vi "configuration UI.vi"() -> ()   [LabVIEW 2018, in "TDMS datalogger editor node.lvclass"]
uses:
  TDMS datalogger editor node.lvclass
  <vilib>/NI/Configuration Framework/Node/NodeRef.ctl
  <vilib>/NI/Configuration Framework/Node/NISE_CEF_Node.lvclass
  <vilib>/NI/AMC/Message Queue.ctl
  <vilib>/NI/AMC/Message.ctl
  <vilib>/NI/Tools/Keyed Array/KeyedArray.ctl
  <vilib>/NI/Configuration Framework/Node/UserEventRef.ctl
  <vilib>/NI/Configuration Framework/Controls/EventCluster.ctl
  <vilib>/NI/DCAF UI Toolkit/Controls/Move One Right.ctl
  <vilib>/NI/DCAF UI Toolkit/Controls/Move All Right.ctl
  <vilib>/NI/DCAF UI Toolkit/Controls/Move One Left.ctl
  <vilib>/NI/Configuration Framework/Node/NodeChangeEvent.ctl
  <vilib>/NI/DCAF UI Toolkit/Controls/Add.ctl
  <vilib>/NI/DCAF UI Toolkit/Controls/Remove.ctl
  <vilib>/NI/Configuration Framework/Node/RefreshUIEvent.ctl
  <vilib>/NI/Configuration Framework/Node/StopEvent.ctl
  <vilib>/NI/Configuration Framework/Node/CacheState.ctl
  <vilib>/NI/DCAF/Tag Editor Core/Table API/Available Tag Menu/channel action event.ctl
  <vilib>/NI/DCAF/Tag Editor Core/Table API/Available Tag Menu/dialog output action.ctl
  <vilib>/NI/Tag Bus Module Framework/channel/TBM channel.lvclass
  <vilib>/NI/Tag Bus/tag/tag descriptor.lvclass
  <vilib>/NI/DCAF/Tag Editor Core/Table API/Table Manager/Call Back Ref Type Def.ctl
  <vilib>/NI/DCAF/Tag Editor Core/Configuration Editor/Classes/Engine Parent/Engine Parent Editor Node.lvclass
  <vilib>/NI/DCAF/Tag Editor Core/Configuration Editor/Classes/Module editor node/module editor node.lvclass
  <vilib>/NI/DCAF UI Toolkit/Controls/Configure.ctl
  <vilib>/NI/DCAF/Tag Editor Core/Table API/Table Manager/object ref.ctl
  <vilib>/NI/DCAF/Tag Editor Core/Table API/Table Manager/references.ctl
  Control Refs.ctl
  <vilib>/Utility/miscctls.llb/LVPositionTypeDef.ctl
  <vilib>/NI/DCAF/Tag Editor Core/Table API/Listbox/Multi Column Listbox.lvclass
  <vilib>/NI/Configuration Framework/NISE_CEF_TreeControl.lvlib
  <vilib>/NI/DCAF UI Toolkit/Controls/DCAF UI Elements.lvlib
  <vilib>/NI/Tools/Keyed Array/Tools_KeyedArray.lvlib
  <vilib>/NI/AMC/AMC.lvlib
  <vilib>/NI/DCAF/Tag Editor Core/Table API/Table Manager/Table Manager.lvclass
  <vilib>/NI/DCAF/Tag Editor Core/Table API/Table Manager.lvlib
panel:
  in  "References":T1
  in  "user event out":refnum<user-event>
  in  "cache state":T2
  in  "stop event":T3
  in  "refresh UI":T4
  in  "node change":T5
  in  "Tab Control":T6(tab)
  in  "channels":i32(listbox)
  in  "remove":T7
  in  "avail tags":i32(listbox)=-1
  in  "add all":T8
  in  "add1":T9
  in  "Use Dynamic File Name":bool
  out "Logging File Path":string
  in  "file name error":bool
  in  "Log Directory":string
  in  "File Name":string
  out "Enable Tag":string
  in  "path error":bool
  in  "Use Enable Channel":bool
  in  "recalc":bool
  out "Approximate Memory Usage":dbl
  in  "Queue Size":u16=2
  in  "Scans Per Write":u16=20
  in  "Log Directory":path
  out "Dynamic File Name Tag":string
  in  "Maximum Age of Files (days)":dbl=365.0
  in  "Rotate count":u32 caption="Maximum Number of Archived Files To Keep"
  in  "archive in place":bool caption="Archive Old Logs in Original Directory"
  in  "Archive Directory":string
  in  "Archive Directory":path
  in  "archive error":bool
  in  "Maximum File Size (KB)":i64=10000
  in  "Channel Subscription Pattern Matches":string[](array[string])
  in  "Enable Dynamic Mapping":bool
  in  "Remove Group":T10
  in  "Add Group":T11
  in  "Remove from Group":T9
  in  "Add to Group":T7
  in  "avail logged tags":i32(listbox)=-1
  in  "Groups":string(tree)="Channel1"
  in  "Add Group Name":string caption="File Name"
  in  "File Property Settings":T12
  in  "File Properties":i32(listbox)=-1
  in  "Add File Property":T11
  in  "Remove File Property":T10
  in  "user event":T13
  in  "main queue":T14
  in  "node ref":T15
  # "kB"
  # "Note: This value ignores dynamic mapping"
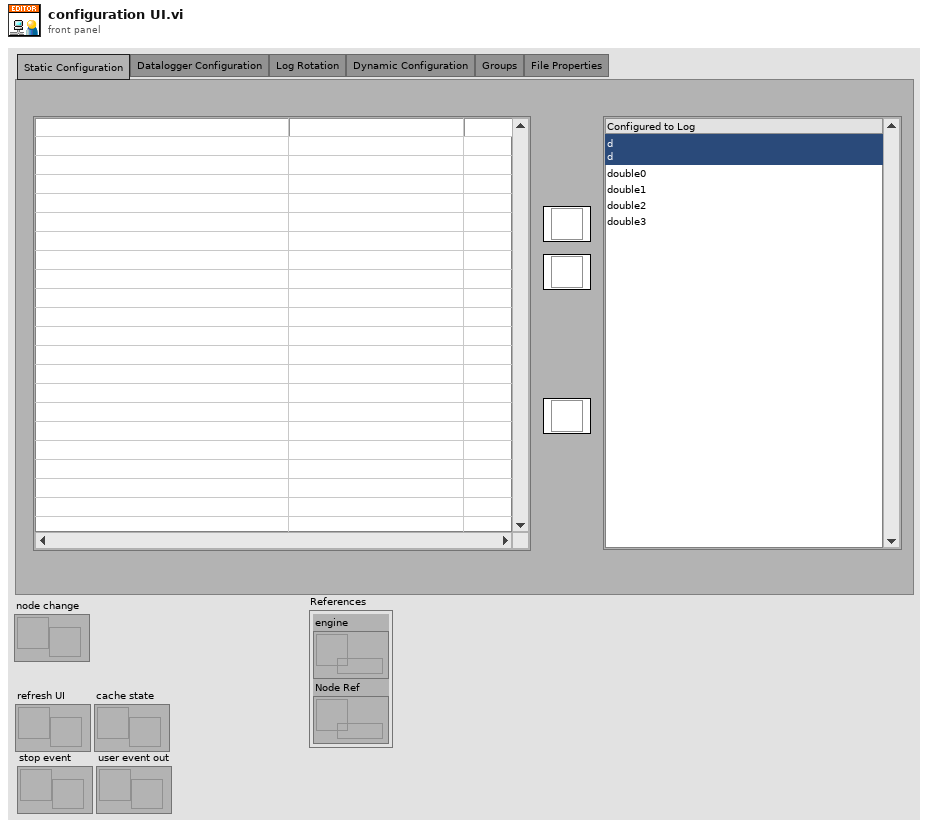
[diagram p1: front panel]
types:
  T1 = typedef "Table Manager.lvlib/Table Manager.lvclass/object ref.ctl" = cluster{"engine":refnum<data-value>, "Node Ref":refnum<data-value>}
  T2 = typedef "NISE_CEF_Node.lvclass/CacheState.ctl" = refnum<user-event>
  T3 = typedef "NISE_CEF_Node.lvclass/StopEvent.ctl" = refnum<user-event>
  T4 = typedef "NISE_CEF_Node.lvclass/RefreshUIEvent.ctl" = refnum<user-event>
  T5 = typedef "NISE_CEF_Node.lvclass/NodeChangeEvent.ctl" = refnum<user-event>
  T6 = enum32{"Static Configuration", "Datalogger Configuration", "Log Rotation", "Dynamic Configuration", "Groups", "File Properties"}
  T7 = typedef "DCAF UI Elements.lvlib/Move One Left.ctl" = bool
  T8 = typedef "DCAF UI Elements.lvlib/Move All Right.ctl" = bool
  T9 = typedef "DCAF UI Elements.lvlib/Move One Right.ctl" = bool
  T10 = typedef "DCAF UI Elements.lvlib/Remove.ctl" = bool
  T11 = typedef "DCAF UI Elements.lvlib/Add.ctl" = bool
  T12 = typedef "DCAF UI Elements.lvlib/Configure.ctl" = bool
  T13 = typedef "NISE_CEF_Node.lvclass/UserEventRef.ctl" = refnum<user-event>
  T14 = typedef "AMC.lvlib/Message Queue.ctl" = refnum<queue>
  T15 = typedef "NISE_CEF_Node.lvclass/NodeRef.ctl" = refnum<data-value>
  T16 = typedef "Control Refs.ctl" = cluster{"avail tags ref":refnum<vi>, "channels ref":refnum<vi>, "File Name ref":refnum<vi>, "Win Log Dir ref":refnum<vi>, "Linux Log Dir ref":refnum<vi>, "Scans Per Write ref":refnum<vi>, "Queue Size ref":refnum<vi>, "Use Enable Channel ref":refnum<vi>, "Maximum File Size ref":refnum<vi>, "Rotate Count ref":refnum<vi>, "Archive in Place ref":refnum<vi>, "Win Archive Dir ref":refnum<vi>, "Linux Archive Dir ref":refnum<vi>, "Max Age ref":refnum<vi>, "Enable Dynamic Mapping ref":refnum<vi>, "Channel Subscription Pattern Matches ref":refnum<vi>, "Add Group Name ref":refnum<vi>, "Groups ref":refnum<vi>, "avail logged tags ref":refnum<vi>, "Archive Error ref":refnum<vi>, "path error ref":refnum<vi>, "file name error ref":refnum<vi>, "Logging File Path":refnum<vi>}
  T17 = typedef "Table Manager.lvlib/Table Manager.lvclass/references.ctl" = cluster{"stop event":T3, "refresh UI":T4, "cache state":T2, "node change":T5, "user event out":refnum<user-event>, "main queue":T14, "user event":T13}
  T18 = typedef "LVPositionTypeDef.ctl" = cluster{"Left":i32, "Top":i32}
  T19 = typedef "Table Manager.lvlib/Column.lvclass/Column Descriptor.ctl" = cluster{"name":string, "caption":string, "Column Type":T20, "Params":string, "AutoSizeMode":i32, "FillWeight":sgl, "MinWidth":u32, "tooltip":string, "Enum Reference":refnum<vi>, "Channel suffix":string, "Read Only":bool, "Call Back VI":T21, "DT Dependency":i32, "name dependency":i32, "data type":T22, "Custom Column":refnum<class "Column.lvclass">}
  T20 = typedef "Table Manager.lvlib/Column.lvclass/Column Type.ctl" = enum16{"String", "Mapping", "Enum", "Custom"}
  T21 = typedef "Table Manager.lvlib/Table Manager.lvclass/Call Back Ref Type Def.ctl" = refnum<vi>
  T22 = typedef "tag bus.lvlib/tag descriptor.lvclass/Data Type.ctl" = enum16{"Double", "Single", "I64", "I32", "I16", "I8", "U64", "U32", "U16", "U8", "Boolean", "String", "Array of Double", "Array of Single", "Array of I64", "Array of I32", "Array of I16", "Array of I8", "Array of U64", "Array of U32", "Array of U16", "Array of U8", "Array of Boolean", "Array of String"}
  T23 = typedef "Table Manager.lvlib/Table Manager.lvclass/Table Events.ctl" = cluster{"Menu Selection":refnum<user-event>}
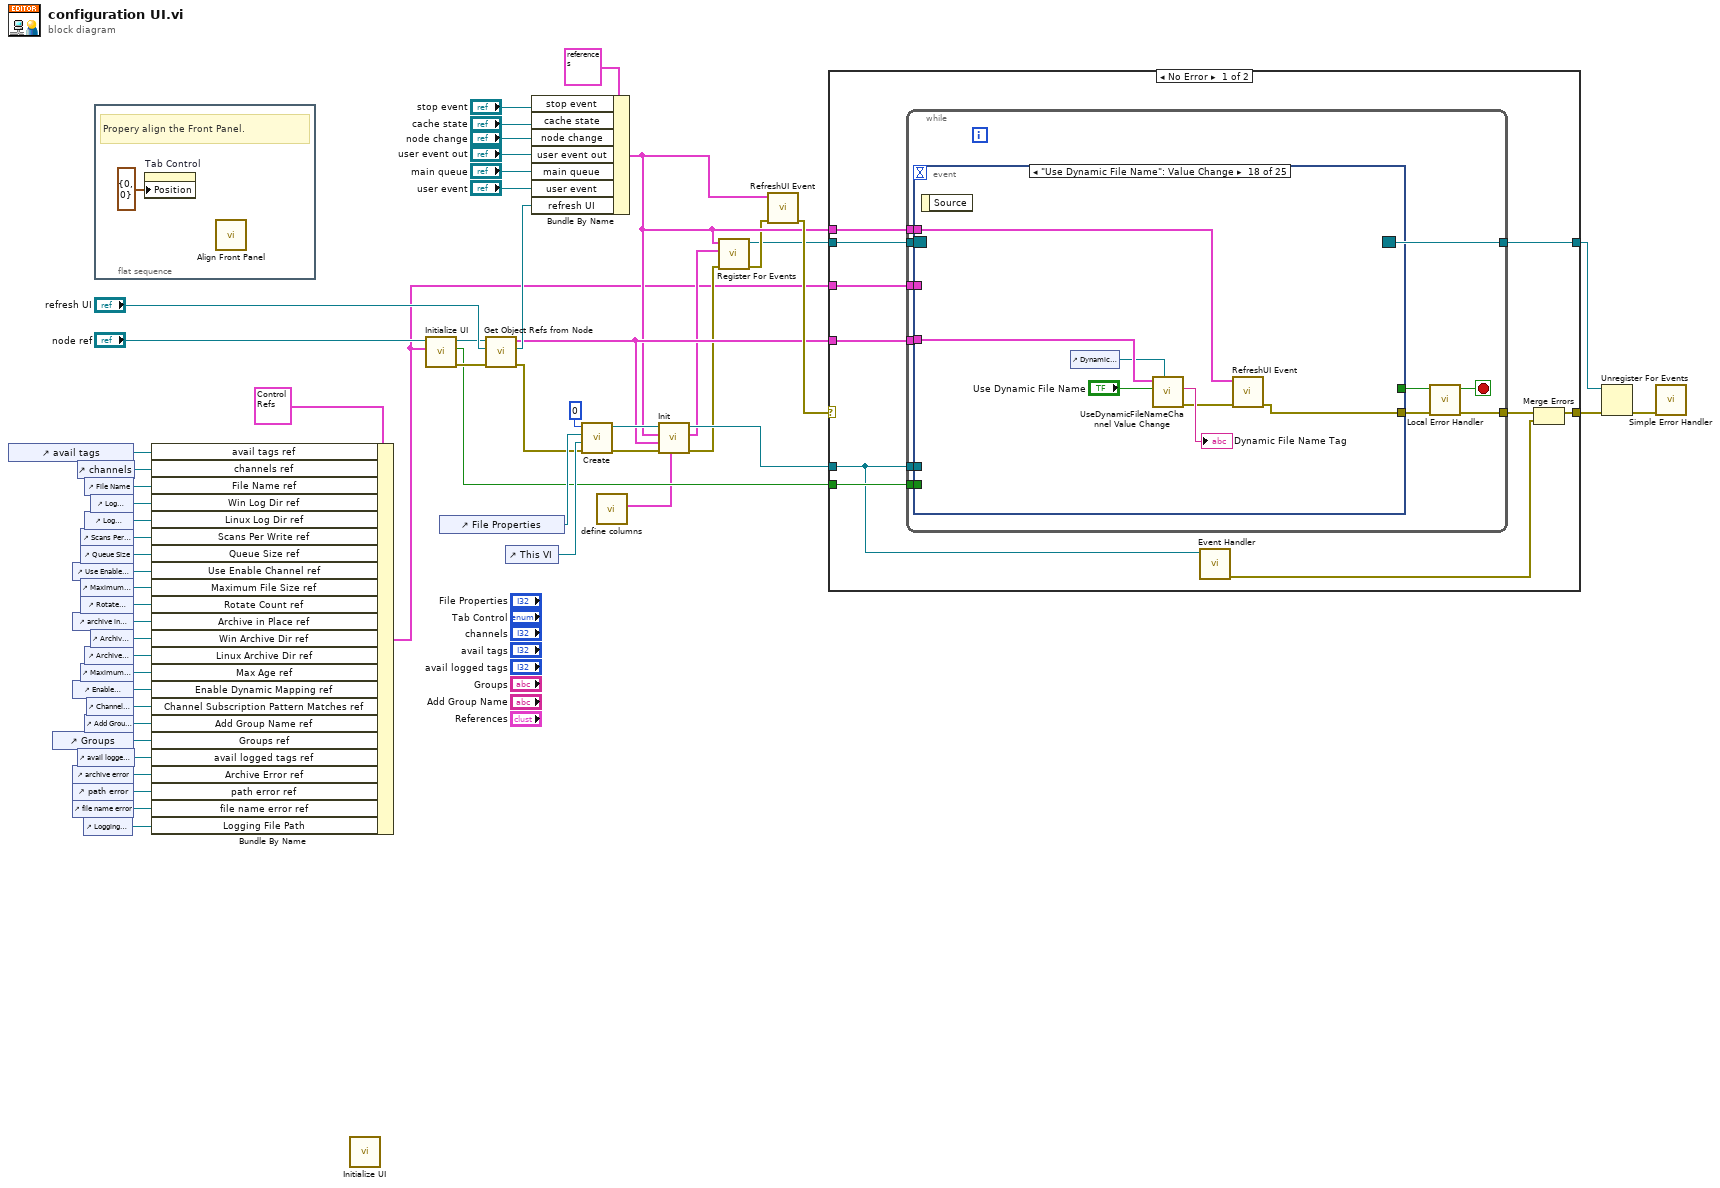
[diagram p0: block diagram]
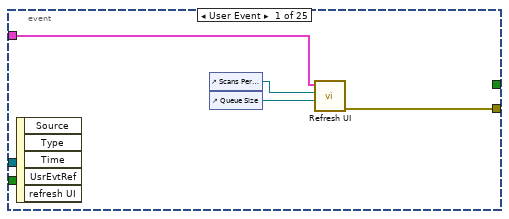
[diagram p2: hidden frame]
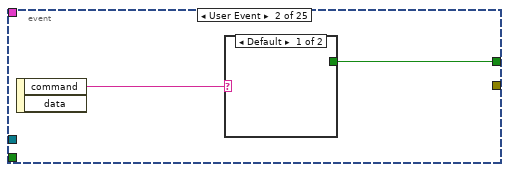
[diagram p3: hidden frame]
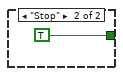
[diagram p4: hidden frame]
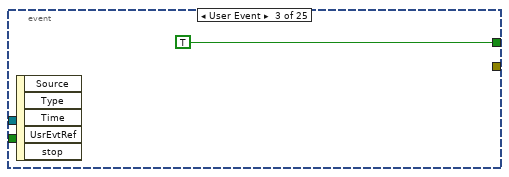
[diagram p5: hidden frame]
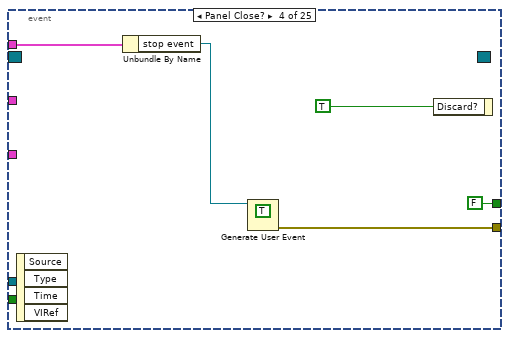
[diagram p6: hidden frame]
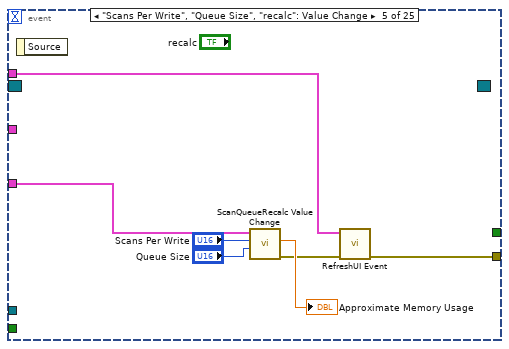
[diagram p7: hidden frame]
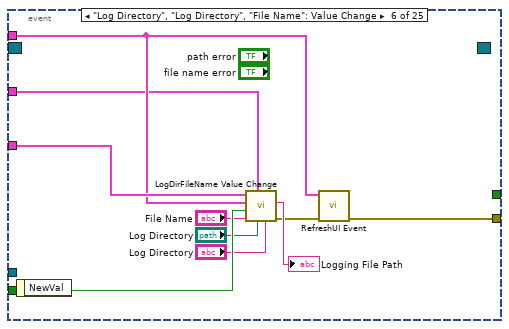
[diagram p8: hidden frame]
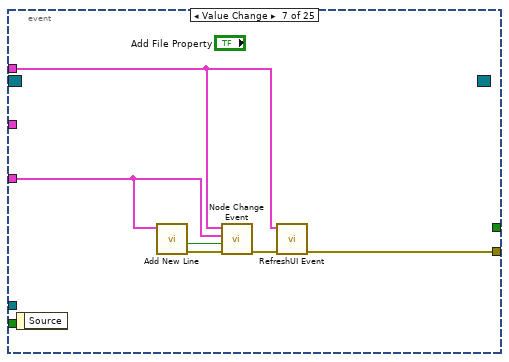
[diagram p9: hidden frame]
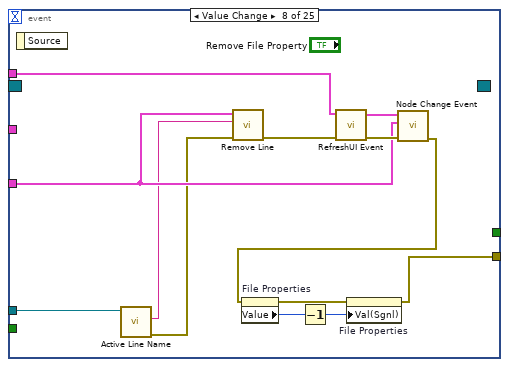
[diagram p10: hidden frame]
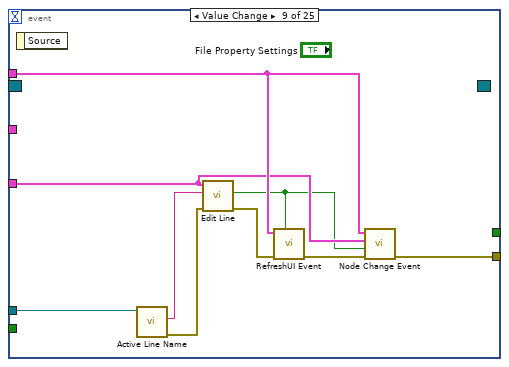
[diagram p11: hidden frame]
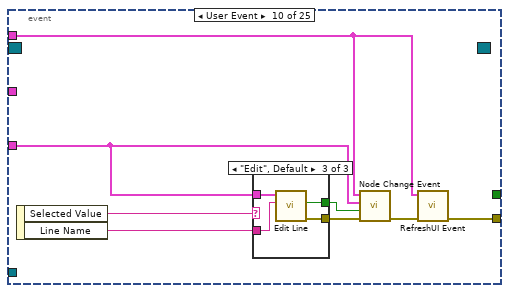
[diagram p12: hidden frame]
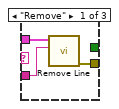
[diagram p13: hidden frame]
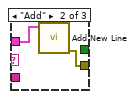
[diagram p14: hidden frame]
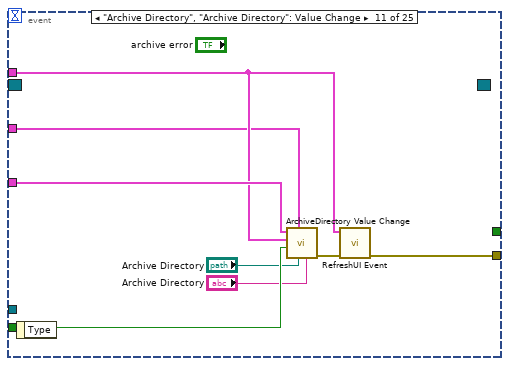
[diagram p15: hidden frame]
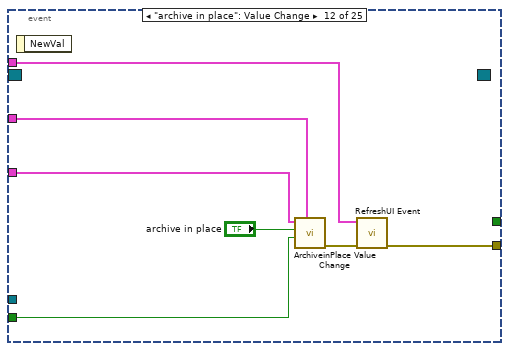
[diagram p16: hidden frame]
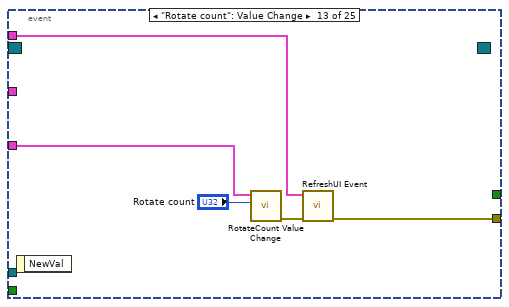
[diagram p17: hidden frame]
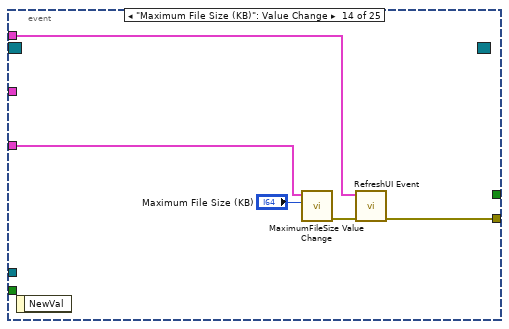
[diagram p18: hidden frame]
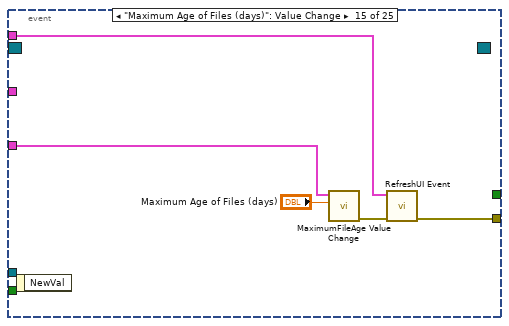
[diagram p19: hidden frame]
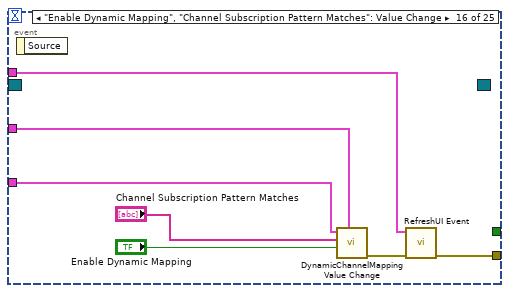
[diagram p20: hidden frame]
diagram:
  n1 = control-ref of="avail tags"() -> (w7:refnum<vi>)
  n2 = control-ref of="Groups"() -> (w24:refnum<vi>)
  n3 = control-ref of="Use Enable Channel"() -> (w14:refnum<vi>)
  n4 = control-ref of="archive in place"() -> (w17:refnum<vi>)
  n5 = control-ref of="Enable Dynamic Mapping"() -> (w21:refnum<vi>)
  n6 = control-ref of="archive error"() -> (w5:refnum<vi>)
  n7 = control-ref of="path error"() -> (w4:refnum<vi>)
  n8 = control-ref of="file name error"() -> (w3:refnum<vi>)
  n9 = control-ref of="channels"() -> (w8:refnum<vi>)
  n10 = control-ref of="avail logged tags"() -> (w25:refnum<vi>)
  n11 = control-ref of="Scans Per Write"() -> (w12:refnum<vi>)
  n12 = control-ref of="Queue Size"() -> (w13:refnum<vi>)
  n13 = control-ref of="Maximum File Size (KB)"() -> (w15:refnum<vi>)
  n14 = control-ref of="Rotate count"() -> (w16:refnum<vi>)
  n15 = control-ref of="Maximum Age of Files (days)"() -> (w20:refnum<vi>)
  n16 = control-ref of="Logging File Path"() -> (w1:refnum<vi>)
  n17 = control-ref of="File Name"() -> (w9:refnum<vi>)
  n18 = control-ref of="Log Directory"() -> (w11:refnum<vi>)
  n19 = control-ref of="Archive Directory"() -> (w19:refnum<vi>)
  n20 = control-ref of="Add Group Name"() -> (w23:refnum<vi>)
  n21 = control-ref of="Channel Subscription Pattern Matches"() -> (w22:refnum<vi>)
  n22 = control-ref of="Log Directory"() -> (w10:refnum<vi>)
  n23 = control-ref of="Archive Directory"() -> (w18:refnum<vi>)
  n24 = flat-sequence {
    frame #0 {
      # "Propery align the Front Panel."
      n25 = property on="Tab Control" class="TabCtl (strict)"("Position"=T18 {"Left"=0, "Top"=0}) -> ()  [unwired: 2 in, 2 out]
      n26 = call <vilib>:"Align Front Panel.vi"() -> ()  [unwired: 10 in, 2 out]
    }
  }
  n27 = Bundle By Name(cluster=T16 {"avail tags ref"=refnum, "channels ref"=refnum, "File Name ref"=refnum, "Win Log Dir ref"=refnum, "Linux Log Dir ref"=refnum, "Scans Per Write ref"=refnum, "Queue Size ref"=refnum, "Use Enable Channel ref"=refnum, "Maximum File Size ref"=refnum, "Rotate Count ref"=refnum, "Archive in Place ref"=refnum, "Win Archive Dir ref"=refnum, "Linux Archive Dir ref"=refnum, "Max Age ref"=refnum, "Enable Dynamic Mapping ref"=refnum, "Channel Subscription Pattern Matches ref"=refnum, "Add Group Name ref"=refnum, "Groups ref"=refnum, "avail logged tags ref"=refnum, "Archive Error ref"=refnum, "path error ref"=refnum, "file name error ref"=refnum, "Logging File Path"=refnum} ("Control Refs"), "avail tags ref"=w7, "channels ref"=w8, "File Name ref"=w9, "Win Log Dir ref"=w10, "Linux Log Dir ref"=w11, "Scans Per Write ref"=w12, "Queue Size ref"=w13, "Use Enable Channel ref"=w14, "Maximum File Size ref"=w15, "Rotate Count ref"=w16, "Archive in Place ref"=w17, "Win Archive Dir ref"=w18, "Linux Archive Dir ref"=w19, "Max Age ref"=w20, "Enable Dynamic Mapping ref"=w21, "Channel Subscription Pattern Matches ref"=w22, "Add Group Name ref"=w23, "Groups ref"=w24, "avail logged tags ref"=w25, "Archive Error ref"=w5, "path error ref"=w4, "file name error ref"=w3, "Logging File Path"=w1) -> (w6:T16)
  n28 = call "Initialize UI.vi"() -> ()  [unwired: 9 in, 3 out]
  n29 = call "Initialize UI.vi"("Control Refs"=w6, "node ref in"="node ref") -> ("error out"=w31:errorcluster, "Linux?"=w28:bool, "node ref out"=w32:T15)  [unwired: 7 in]
  n30 = control-ref of="File Properties"() -> (w38:refnum<vi>)
  n31 = call "Get Object Refs from Node.vi"("error in (no error)"=w31, "Refresh UI"="refresh UI", "node ref"=w32) -> ("error out"=w30:errorcluster, "Refresh UI out"=w40:T4, "References"=w39:T1)  [unwired: 6 in]
  n32 = control-ref of="This VI"() -> (w45:refnum<vi>)
  n33 = Bundle By Name(cluster=T17 {"stop event"=refnum, "refresh UI"=refnum, "cache state"=refnum, "node change"=refnum, "user event out"=refnum, "main queue"=refnum, "user event"=refnum} ("References"), "stop event"="stop event", "cache state"="cache state", "node change"="node change", "user event out"="user event out", "main queue"="main queue", "user event"="user event", "refresh UI"=w40) -> (w37:T17)
  n34 = call <vilib>:"Create.vi"("error in (no error)"=w30, "Top VI"=w45, "Listbox"=w38, "Index"=0) -> ("error out"=w43:errorcluster, "reference out"=w44:refnum<class "Multi Column Listbox.lvclass">)  [unwired: 6 in]
  n35 = call "define columns.vi"() -> ("Column Definition"=w2:T19[])  [unwired: 11 in]
  n36 = call-dynamic "Init.vi"("Column Descriptors"=w2, "error in (no error)"=w43, "Node object refs"=w39, "Event References"=w37, "Multi Column Listbox in"=w44) -> ("error out"=w29:errorcluster, "Table Events"=w27:T23, "Multi Column Listbox out"=w41:refnum<class "Multi Column Listbox.lvclass">)  [unwired: 4 in]
  n37 = call "Register For Events.vi"("error in"=w29, "Table Events"=w27, "References"=w37) -> ("error out"=w36:errorcluster, "Event Registration Refnum"=w35:refnum<event-registration>)  [unwired: 7 in]
  n38 = call "RefreshUI Event.vi"("error in (no error)"=w36, "References in"=w37) -> ("error out"=w42:errorcluster)  [unwired: 8 in, 1 out]
  n39 = case shown="No Error" w42 {
    selector: w42 -> [_ w239]
    tunnel: w35 -> [w67 w238]
    tunnel: [w66 w238] -> w56
    tunnel: [w60 w239] -> w54
    tunnel: w28 -> [w64 _]
    tunnel: w39 -> [w63 _]
    tunnel: w41 -> [w62 _]
    tunnel: w37 -> [w61 _]
    tunnel: w6 -> [w58 _]
    frame No Error {
      n40 = while {
        tunnel: w67 -> [w78]
        tunnel: [w77] -> w66
        tunnel: [w72] -> w65
        tunnel: w64 -> [w76]
        tunnel: w63 -> [w68]
        tunnel: w62 -> [w75]
        tunnel: w61 -> [w74]
        tunnel: w58 -> [w69]
        stop <- w70 stop-if-true
        n41 = event shown="[17] \"Use Dynamic File Name\": Value Change" {
          selector: w78 -> [_ _ _ _ _ _ _ _ _ _ _ _ _ _ _ _ _ _ _ _ _ _ _ _ _]
          dyn-events: [_ _ _ _ _ _ _ _ _ _ _ _ _ _ _ _ _ _ _ _ _ _ _ _ _] -> w77
          timeout: _ -> [_ _ _ _ _ _ _ _ _ _ _ _ _ _ _ _ _ _ _ _ _ _ _ _ _]
          tunnel: [_ w83 TRUE FALSE _ _ _ _ _ _ _ _ _ _ _ _ _ _ _ _ _ _ _ _ _] -> w71
          tunnel: [w81 _ _ w91 w94 w101 w112 w124 w129 w143 w162 w164 w171 w176 w180 w189 w192 w200 w206 w211 w215 w218 w222 w226 w234] -> w73
          tunnel: w76 -> [_ _ _ _ _ w107 _ _ _ _ w159 w168 _ _ _ _ _ _ _ _ _ _ _ _ _]
          tunnel: w68 -> [w82 _ _ _ w98 w109 w110 w119 w131 w138 w161 w167 w173 w178 w182 w187 w197 w205 w208 w210 w216 w220 w224 w228 w233]
          tunnel: w75 -> [_ _ _ _ _ _ _ w128 w137 _ _ _ _ _ _ _ _ _ _ _ _ _ _ _ _]
          tunnel: w74 -> [_ _ _ w90 w99 w108 w111 w122 w132 w139 w160 w169 w174 w175 w184 w191 w198 w199 w209 w213 w217 w221 w225 w229 w237]
          tunnel: w69 -> [_ _ _ _ _ w100 _ _ _ _ w155 w163 _ _ _ w185 _ _ _ _ _ _ _ _ _]
          event User Event {
            n42 = event-data() -> ()  [unwired: 1 in, 5 out]
            n43 = control-ref of="Scans Per Write"() -> (w80:refnum<vi>)
            n44 = control-ref of="Queue Size"() -> (w79:refnum<vi>)
            n45 = call "Refresh UI.vi"("Queue Size ref"=w79, "Scans Per Write ref"=w80, "References"=w82) -> ("error out"=w81:errorcluster)  [unwired: 8 in]
          }
          event User Event {
            n46 = event-data() -> ("command"=w84:string)  [unwired: 1 in, 1 out]
            n47 = case shown="Default" w84 {
              tunnel: [_ TRUE] -> w83
              frame Default {
              }
              frame "Stop" {
              }
            }
          }
          event User Event {
            n48 = event-data() -> ()  [unwired: 1 in, 5 out]
          }
          event Panel Close? {
            n49 = event-data() -> ()  [unwired: 1 in, 4 out]
            n50 = Unbundle By Name(w90) -> ("stop event"=w89:T3)
            n51 = Generate User Event(user event=w89, event data cluster=TRUE ("event data")) -> (error out=w91:errorcluster)  [unwired: 2 in, 1 out]
            n52 = event-data("Discard?"=TRUE) -> ()  [unwired: 1 in, 1 out]
          }
          event "Scans Per Write", "Queue Size", "recalc": Value Change {
            n53 = event-data() -> ()  [unwired: 1 in, 1 out]
            n54 = call "ScanQueueRecalc Value Change.vi"("Queue Size"="Queue Size", "Scans Per Write"="Scans Per Write", "References"=w98) -> ("error out"=w93:errorcluster, "Approximate Memory Usage"=→"Approximate Memory Usage":dbl)  [unwired: 7 in]
            n55 = call "RefreshUI Event.vi"("error in (no error)"=w93, "References in"=w99) -> ("error out"=w94:errorcluster)  [unwired: 8 in, 1 out]
          }
          event "Log Directory", "Log Directory", "File Name": Value Change {
            n56 = event-data() -> ()  [unwired: 1 in, 1 out]
            n57 = call "LogDirFileName Value Change.vi"("Linux Log Directory"="Log Directory", "Windows Log Directory"="Log Directory", "Control Refs"=w100, "File Name"="File Name", "Linux Paths?"=w107, "Event References"=w108, "References"=w109) -> ("error out"=w102:errorcluster, "Logging File Path"=→"Logging File Path":string)  [unwired: 3 in]
            n58 = call "RefreshUI Event.vi"("error in (no error)"=w102, "References in"=w108) -> ("error out"=w101:errorcluster)  [unwired: 8 in, 1 out]
          }
          event Value Change {
            n59 = event-data() -> ()  [unwired: 1 in, 1 out]
            n60 = call "Add New Line.vi"("objects"=w110) -> ("error out"=w115:errorcluster, "success"=w114:bool)  [unwired: 8 in, 1 out]
            n61 = call "Node Change Event.vi"("error in (no error)"=w115, "Send (T)"=w114, "objects"=w110, "References in"=w111) -> ("error out"=w113:errorcluster)  [unwired: 7 in]
            n62 = call "RefreshUI Event.vi"("error in (no error)"=w113, "References in"=w111) -> ("error out"=w112:errorcluster)  [unwired: 8 in, 1 out]
          }
          event Value Change {
            n63 = event-data() -> ()  [unwired: 1 in, 1 out]
            n64 = call-dynamic "Active Line Name.vi"("Multi Column Listbox in"=w128) -> ("error out"=w116:errorcluster, "Active Line Name"=w118:string)  [unwired: 8 in, 1 out]
            n65 = call "Remove Line.vi"("error in"=w116, "Active Line Name"=w118, "Objects"=w119) -> ("error out"=w117:errorcluster)  [unwired: 8 in]
            n66 = call "RefreshUI Event.vi"("error in (no error)"=w117, "References in"=w122) -> ("error out"=w123:errorcluster, "References out"=w121:T17)  [unwired: 8 in]
            n67 = call "Node Change Event.vi"("error in (no error)"=w123, "objects"=w119, "References in"=w121) -> ("error out"=w120:errorcluster)  [unwired: 8 in]
            n68 = property on="File Properties" class="MCListbox (strict)"(error in=w120) -> (error out=w125:errorcluster, "Value"=w127:i32)  [unwired: 1 in, 1 out]
            n69 = Decrement(x=w127) -> (x-1=w126:i32)
            n70 = property on="File Properties" class="MCListbox (strict)"(error in=w125, "Val(Sgnl)"=w126) -> (error out=w124:errorcluster)  [unwired: 1 in, 1 out]
          }
          event Value Change {
            n71 = event-data() -> ()  [unwired: 1 in, 1 out]
            n72 = call-dynamic "Active Line Name.vi"("Multi Column Listbox in"=w137) -> ("error out"=w136:errorcluster, "Active Line Name"=w135:string)  [unwired: 8 in, 1 out]
            n73 = call "Edit Line.vi"("error in"=w136, "Line Name"=w135, "References"=w131) -> ("error out"=w134:errorcluster, "change?"=w130:bool)  [unwired: 7 in]
            n74 = call "RefreshUI Event.vi"("Refresh (T)"=w130, "error in (no error)"=w134, "References in"=w132) -> ("error out"=w133:errorcluster)  [unwired: 7 in, 1 out]
            n75 = call "Node Change Event.vi"("error in (no error)"=w133, "Send (T)"=w130, "objects"=w131, "References in"=w132) -> ("error out"=w129:errorcluster)  [unwired: 7 in]
          }
          event User Event {
            n76 = event-data() -> ("Selected Value"=w145:string, "Line Name"=w144:string)  [unwired: 1 in]
            n77 = case shown="\"Edit\", Default" w145 {
              tunnel: w144 -> [w146 _ w151]
              tunnel: w138 -> [w147 w149 w153]
              tunnel: [w148 w150 w154] -> w141
              tunnel: [_ _ w152] -> w140
              frame "Remove" {
                n78 = call "Remove Line.vi"("Active Line Name"=w146, "Objects"=w147) -> ("error out"=w148:errorcluster)  [unwired: 9 in]
              }
              frame "Add" {
                n79 = call "Add New Line.vi"("objects"=w149) -> ("error out"=w150:errorcluster)  [unwired: 8 in, 2 out]
              }
              frame "Edit", Default {
                n80 = call "Edit Line.vi"("Line Name"=w151, "References"=w153) -> ("error out"=w154:errorcluster, "change?"=w152:bool)  [unwired: 8 in]
              }
            }
            n81 = call "Node Change Event.vi"("error in (no error)"=w141, "Send (T)"=w140, "objects"=w138, "References in"=w139) -> ("error out"=w142:errorcluster)  [unwired: 7 in]
            n82 = call "RefreshUI Event.vi"("error in (no error)"=w142, "References in"=w139) -> ("error out"=w143:errorcluster)  [unwired: 8 in, 1 out]
          }
          event "Archive Directory", "Archive Directory": Value Change {
            n83 = event-data() -> ()  [unwired: 1 in, 1 out]
            n84 = call "ArchiveDirectory Value Change.vi"("Linux Archive Directory"="Archive Directory", "Windows Archive Directory"="Archive Directory", "Control Refs"=w155, "Linux Paths?"=w159, "Event References"=w160, "References"=w161) -> ("error out"=w156:errorcluster)  [unwired: 5 in]
            n85 = call "RefreshUI Event.vi"("error in (no error)"=w156, "References in"=w160) -> ("error out"=w162:errorcluster)  [unwired: 8 in, 1 out]
          }
          event "archive in place": Value Change {
            n86 = event-data() -> ()  [unwired: 1 in, 1 out]
            n87 = call "ArchiveinPlace Value Change.vi"("Control Refs"=w163, "Linux?"=w168, "archive in place"="archive in place", "References"=w167) -> ("error out"=w165:errorcluster)  [unwired: 7 in]
            n88 = call "RefreshUI Event.vi"("error in (no error)"=w165, "References in"=w169) -> ("error out"=w164:errorcluster)  [unwired: 8 in, 1 out]
          }
          event "Rotate count": Value Change {
            n89 = event-data() -> ()  [unwired: 1 in, 1 out]
            n90 = call "RotateCount Value Change.vi"("Rotate count"="Rotate count", "References"=w173) -> ("error out"=w172:errorcluster)  [unwired: 9 in]
            n91 = call "RefreshUI Event.vi"("error in (no error)"=w172, "References in"=w174) -> ("error out"=w171:errorcluster)  [unwired: 8 in, 1 out]
          }
          event "Maximum File Size (KB)": Value Change {
            n92 = event-data() -> ()  [unwired: 1 in, 1 out]
            n93 = call "MaximumFileSize Value Change.vi"("Maximum File Size (KB)"="Maximum File Size (KB)", "References"=w178) -> ("error out"=w177:errorcluster)  [unwired: 9 in]
            n94 = call "RefreshUI Event.vi"("error in (no error)"=w177, "References in"=w175) -> ("error out"=w176:errorcluster)  [unwired: 8 in, 1 out]
          }
          event "Maximum Age of Files (days)": Value Change {
            n95 = event-data() -> ()  [unwired: 1 in, 1 out]
            n96 = call "MaximumFileAge Value Change.vi"("Maximum Age of Files (days)"="Maximum Age of Files (days)", "References"=w182) -> ("error out"=w181:errorcluster)  [unwired: 9 in]
            n97 = call "RefreshUI Event.vi"("error in (no error)"=w181, "References in"=w184) -> ("error out"=w180:errorcluster)  [unwired: 8 in, 1 out]
          }
          event "Enable Dynamic Mapping", "Channel Subscription Pattern Matches": Value Change {
            n98 = event-data() -> ()  [unwired: 1 in, 1 out]
            n99 = call "DynamicChannelMapping Value Change.vi"("Control Refs"=w185, "Enable Dynamic Mapping"="Enable Dynamic Mapping", "Channel Subscription Pattern Matches"="Channel Subscription Pattern Matches", "References"=w187) -> ("error out"=w190:errorcluster)  [unwired: 7 in]
            n100 = call "RefreshUI Event.vi"("error in (no error)"=w190, "References in"=w191) -> ("error out"=w189:errorcluster)  [unwired: 8 in, 1 out]
          }
          event "Use Enable Channel": Value Change {
            n101 = event-data() -> ()  [unwired: 1 in, 1 out]
            n102 = control-ref of="Enable Tag"() -> (w195:refnum<vi>)
            n103 = call "UseEnableChannel Value Change.vi"("Enable Tag ref"=w195, "Use Enable Channel"="Use Enable Channel", "References"=w197) -> ("error out"=w193:errorcluster, "Enable Tag"=→"Enable Tag":string)  [unwired: 7 in]
            n104 = call "RefreshUI Event.vi"("error in (no error)"=w193, "References in"=w198) -> ("error out"=w192:errorcluster)  [unwired: 8 in, 1 out]
          }
          event "Use Dynamic File Name": Value Change {
            n105 = event-data() -> ()  [unwired: 1 in, 1 out]
            n106 = control-ref of="Dynamic File Name Tag"() -> (w204:refnum<vi>)
            n107 = call "UseDynamicFileNameChannel Value Change.vi"("Dynamic File Name Tag ref"=w204, "Use Dynamic File Name"="Use Dynamic File Name", "References"=w205) -> ("error out"=w201:errorcluster, "Dynamic File Name Tag"=→"Dynamic File Name Tag":string)  [unwired: 7 in]
            n108 = call "RefreshUI Event.vi"("error in (no error)"=w201, "References in"=w199) -> ("error out"=w200:errorcluster)  [unwired: 8 in, 1 out]
          }
          event Value Change {
            n109 = event-data() -> ()  [unwired: 1 in, 1 out]
            n110 = call "Add1 Value Change.vi"("References"=w208) -> ("error out"=w207:errorcluster)  [unwired: 10 in]
            n111 = call "RefreshUI Event.vi"("error in (no error)"=w207, "References in"=w209) -> ("error out"=w206:errorcluster)  [unwired: 8 in, 1 out]
          }
          event Value Change {
            n112 = event-data() -> ()  [unwired: 1 in, 1 out]
            n113 = call "AddGroup Value Change.vi"("References"=w210) -> ("error out"=w212:errorcluster)  [unwired: 10 in]
            n114 = call "RefreshUI Event.vi"("error in (no error)"=w212, "References in"=w213) -> ("error out"=w211:errorcluster)  [unwired: 8 in, 1 out]
          }
          event Value Change {
            n115 = event-data() -> ()  [unwired: 1 in, 1 out]
            n116 = call "RemoveGroup Value Change.vi"("References"=w216) -> ("error out"=w214:errorcluster)  [unwired: 10 in]
            n117 = call "RefreshUI Event.vi"("error in (no error)"=w214, "References in"=w217) -> ("error out"=w215:errorcluster)  [unwired: 8 in, 1 out]
          }
          event Value Change {
            n118 = event-data() -> ()  [unwired: 1 in, 1 out]
            n119 = call "RemoveFromGroup Value Change.vi"("References"=w220) -> ("error out"=w219:errorcluster)  [unwired: 10 in]
            n120 = call "RefreshUI Event.vi"("error in (no error)"=w219, "References in"=w221) -> ("error out"=w218:errorcluster)  [unwired: 8 in, 1 out]
          }
          event Value Change {
            n121 = event-data() -> ()  [unwired: 1 in, 1 out]
            n122 = call "AddToGroup Value Change.vi"("References"=w224) -> ("error out"=w223:errorcluster)  [unwired: 10 in]
            n123 = call "RefreshUI Event.vi"("error in (no error)"=w223, "References in"=w225) -> ("error out"=w222:errorcluster)  [unwired: 8 in, 1 out]
          }
          event Value Change {
            n124 = event-data() -> ()  [unwired: 1 in, 1 out]
            n125 = call "AddAll Value Change.vi"("References"=w228) -> ("error out"=w227:errorcluster)  [unwired: 10 in]
            n126 = call "RefreshUI Event.vi"("error in (no error)"=w227, "References in"=w229) -> ("error out"=w226:errorcluster)  [unwired: 8 in, 1 out]
          }
          event Value Change {
            n127 = event-data() -> ()  [unwired: 1 in, 1 out]
            n128 = local read "channels"() -> (w236:i32)
            n129 = call "RemoveChannel Value Change.vi"("channel"=w236, "References"=w233) -> ("error out"=w235:errorcluster, "Removed Channel Name"=w232:string)  [unwired: 8 in]
            n130 = call "Remove Unlogged Channel from Group.vi"("Item Name"=w232, "References"=w233) -> ("error out"=w230:errorcluster)  [unwired: 9 in]
            n131 = Merge Errors(w230, w235) -> (w231:errorcluster)
            n132 = call "RefreshUI Event.vi"("error in (no error)"=w231, "References in"=w237) -> ("error out"=w234:errorcluster)  [unwired: 8 in, 1 out]
          }
        }
        n133 = call "Local Error Handler.vi"("error in"=w73, "Stop in"=w71) -> ("error out"=w72:errorcluster, "Stop out"=w70:bool)  [unwired: 8 in]
      }
      n134 = call-dynamic "Event Handler.vi"("Listbox in"=w62) -> ("error out"=w59:errorcluster)  [unwired: 9 in, 1 out]
      n135 = Merge Errors(w65, w59) -> (w60:errorcluster)
    }
    frame Error {
    }
  }
  n136 = Unregister For Events(event registration refnum=w56, error in=w54) -> (error out=w55:errorcluster)
  n137 = call <vilib>:"Simple Error Handler.vi"("error in (no error)"=w55) -> ()  [unwired: 4 in, 5 out]
